vi "FeedbackDecode_Str2Num.vi"(1 "InputString":string caption="Input String") -> (0 "Array":dbl[](array[numeric]))   [LabVIEW 2020]
uses:
  <vilib>/regexp/Match Regular Expression.xnode
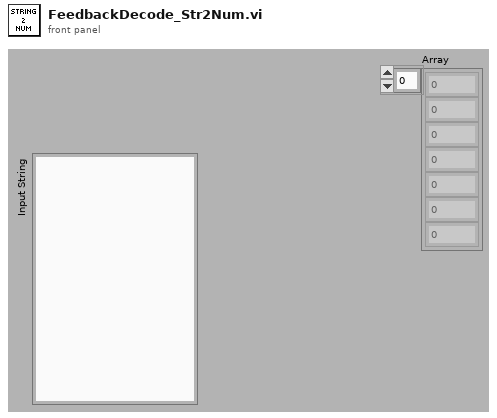
[diagram p1: front panel]
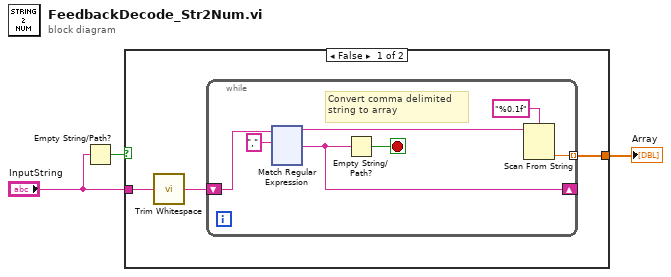
[diagram p0: block diagram]
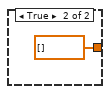
[diagram p2: hidden frame]
diagram:
  n1 = Empty String/Path?(string/path="InputString") -> (empty?=w2:bool)
  n2 = case shown="False" w2 {
    tunnel: "InputString" -> [w6 _]
    tunnel: [w4 dbl[] []] -> w3
    frame False {
      n3 = call <vilib>:"Trim Whitespace.vi"("string"=w6) -> ("trimmed string"=w5:string)  [unwired: 1 in]
      n4 = while {
        shift-right: [w8] -> _
        shift-left: w5 -> [w12]
        tunnel: [w10] -> w4 mode=indexing
        stop <- w7 stop-if-true
        # "Convert comma delimited\nstring to array"
        n5 = xnode "Match Regular Expression"("input string"=w12, "regular expression"=",") -> ("before match"=w11:string, "after match"=w8:string)  [unwired: 4 in, 3 out]
        n6 = Empty String/Path?(string/path=w8) -> (empty?=w7:bool)
        n7 = Scan From String(format string="%0.1f", input string=w11) -> (output 1=w10:dbl)  [unwired: 3 in, 3 out]
      }
    }
    frame True {
    }
  }
  "Array" <- w3
